vi "WriteCal.vi"(11 "Calibration table":T1={"version"=3, "table type"=25, "table size"=496, "full version"=67109889, "crc32"=2980334277, "baseline"=-55.153587, "model"=1, "fx left"=0.7094939, "fy left"=1.2617997, "px left"=0.49358395, "py left"=0.4803248, "py right"=0.4684578, "px right"=0.4979801, "fy right"=1.2668592, "fx right"=0.7124277, "k left"=[0.13808699, -0.41154006, 0.00043059044, 0.00047021545, 0.34858656], "k right"=[0.14090613, -0.42654052, -0.0003404384, 0.0005577445, 0.36482877], "RLeft"=[0.99998826, -0.004810224, 0.0006247892, 0.0048055355, 0.9999618, 0.0073000034, -0.00065988, -0.007296915, 0.9999732], "Rright"=[0.9999898, 0.00018351649, -0.0045086313, -0.00021641784, 0.99997336, -0.0072980113, 0.004507172, 0.007298913, 0.9999632], "uint8 reserved1"=[0, 0, 0, 0, 0, 0, 0, 0, 0, 0, 0, 0, 0, 0, 0, 0, 0, 0, 0, 0, 0, 0, 0, 0, 0, 0, 0, 0, 0, 0, 0, 0, 0, 0, 0, 0, 0, 0, 0, 0, 0, 0, 0, 0, 0, 0, 0, 0, 0, 0, 0, 0, 0, 0, 0, 0, 0, 0, 0, 0, 0, 0, 0, 0, 0, 0, 0, 0, 0, 0, 0, 0, 0, 0, 0, 0, 0, 0, 0, 0, 0, 0, 0, 0, 0, 0, 0, 0], "uint8 reserved2"=[0, 0, 0, 0, 0, 0, 0, 0, 0, 0, 0, 0, 0, 0, 0, 0, 0, 0, 0, 0, 0, 0, 0, 0, 0, 0, 0, 0, 0, 0, 0, 0, 0, 0, 0, 0, 0, 0, 0, 0, 0, 0, 0, 0, 0, 0, 0, 0, 0, 0, 0, 0, 0, 0, 0, 0, 0, 0, 0, 0, 0, 0, 0, 0], "1920x1080"=[1442.0812, 1442.0812, 949.4115, 513.11053], "1280x720"=[961.38745, 961.38745, 632.941, 342.07367], "640x480"=[640.925, 640.925, 315.29398, 228.04912], "848x480"=[640.925, 640.925, 419.29398, 228.04912], "640x360"=[480.69373, 480.69373, 316.4705, 171.03683], "424x240"=[320.4625, 320.4625, 209.64699, 114.02456], "320x240"=[320.4625, 320.4625, 157.64699, 114.02456], "480x270"=[360.5203, 360.5203, 237.35287, 128.27763], "1280x800"=[1068.2083, 1068.2083, 632.1567, 380.08188], "960x540"=[721.0406, 721.0406, 474.70575, 256.55527], "Reserved1"=[0.0, 0.0, 0.0, 0.0], "Reserved 2"=[0.0, 0.0, 0.0, 0.0]} {"crc32" format="%x"}) -> (2 "size":i32=512, 3 "Output array":u8[](array[numeric])=[197, 74, 164, 177, 240, 1, 0, 0, 1, 4, 0, 4, 197, 74, 164, 177, 100, 161, 53, 63, 167, 130, 161, 63, 9, 183, 252, 62, 34, 237, 245, 62, 173, 102, 13, 62, 97, 181, 210, 190, 223, 192, 225, 57, 64, 135, 246, 57, 240, 121, 178, 62, 169, 97, 54, 63, 113, 40, 162, 63, 63, 247, 254, 62, 179, 217, 239, 62, 178, 73, 16, 62, 133, 99, 218, 190, 222, 124, 178, 185, 154, 53, 18, 58, 214, 202, 186, 62, 59, 255, 127, 63, 21, 159, 157, 187, 229, 200, 35, 58, 193, 119, 157, 59, 127, 253, 127, 63, 222, 52, 239, 59, 204, 251, 44, 186, 246, 26, 239, 187, 62, 254, 127, 63, 85, 255, 127, 63, 85, 110, 64, 57, 36, 189, 147, 187, 57, 238, 98, 185, 65, 254, 127, 63, 40, 36, 239, 187, 230, 176, 147, 59, 184, 43, 239, 59, 151, 253, 127, 63, 70, 157, 92, 194, 1, 0, 0, 0, 0, 0, 0, 0, 0, 0, 0, 0, 0, 0, 0, 0, 0, 0, 0, 0, 0, 0, 0, 0, 0, 0, 0, 0, 0, 0, 0, 0, 0, 0, 0, 0, 0, 0, 0, 0, 0, 0, 0, 0, 0, 0, 0, 0, 0, 0, 0, 0, 0, 0, 0, 0, 0, 0, 0, 0, 0, 0, 0, 0, 0, 0, 0, 0, 0, 0, 0, 0, 0, 0, 0, 0, 0, 0, 0, 0, 0, 0, 0, 0, 0, 0, 0, 0, 0, 0, 0, 0, 153, 66, 180, 68, 153, 66, 180, 68, 86, 90, 109, 68, 19, 71, 0, 68, 204, 88, 112, 68, 204, 88, 112, 68, 57, 60, 30, 68, 110, 9, 171, 67, 51, 59, 32, 68, 51, 59, 32, 68, 161, 165, 157, 67, 147, 12, 100, 67, 51, 59, 32, 68, 51, 59, 32, 68, 161, 165, 209, 67, 147, 12, 100, 67, 204, 88, 240, 67, 204, 88, 240, 67, 57, 60, 158, 67, 110, 9, 43, 67, 51, 59, 160, 67, 51, 59, 160, 67, 161, 165, 81, 67, 147, 12, 228, 66, 51, 59, 160, 67, 51, 59, 160, 67, 161, 165, 29, 67, 147, 12, 228, 66, 153, 66, 180, 67, 153, 66, 180, 67, 86, 90, 109, 67, 19, 71, 0, 67, 170, 134, 133, 68, 170, 134, 133, 68, 7, 10, 30, 68, 123, 10, 190, 67, 153, 66, 52, 68, 153, 66, 52, 68, 86, 90, 237, 67, 19, 71, 128, 67, 0, 0, 0, 0, 0, 0, 0, 0, 0, 0, 0, 0, 0, 0, 0, 0, 0, 0, 0, 0, 0, 0, 0, 0, 0, 0, 0, 0, 0, 0, 0, 0, 0, 0, 0, 0, 0, 0, 0, 0, 0, 0, 0, 0, 0, 0, 0, 0, 0, 0, 0, 0, 0, 0, 0, 0, 0, 0, 0, 0, 0, 0, 0, 0, 0, 0, 0, 0, 0, 0, 0, 0, 0, 0, 0, 0, 0, 0, 0, 0, 0, 0, 0, 0, 0, 0, 0, 0, 0, 0, 0, 0, 0, 0, 0, 0] format="%x")   [LabVIEW 2017, in "libRealSense3.lvlib"]
uses:
  libRealSense3.lvlib
panel:
  out "input":u8[](array[numeric]) format="%x"
  out "Calibration table 2":T1={"version"=3, "table type"=25, "table size"=496, "full version"=67109889, "crc32"=2980334277, "baseline"=-55.153587, "model"=1, "fx left"=0.7094939, "fy left"=1.2617997, "px left"=0.49358395, "py left"=0.4803248, "py right"=0.4684578, "px right"=0.4979801, "fy right"=1.2668592, "fx right"=0.7124277, "k left"=[0.13808699, -0.41154006, 0.00043059044, 0.00047021545, 0.34858656], "k right"=[0.14090613, -0.42654052, -0.0003404384, 0.0005577445, 0.36482877], "RLeft"=[0.99998826, -0.004810224, 0.0006247892, 0.0048055355, 0.9999618, 0.0073000034, -0.00065988, -0.007296915, 0.9999732], "Rright"=[0.9999898, 0.00018351649, -0.0045086313, -0.00021641784, 0.99997336, -0.0072980113, 0.004507172, 0.007298913, 0.9999632], "uint8 reserved1"=[0, 0, 0, 0, 0, 0, 0, 0, 0, 0, 0, 0, 0, 0, 0, 0, 0, 0, 0, 0, 0, 0, 0, 0, 0, 0, 0, 0, 0, 0, 0, 0, 0, 0, 0, 0, 0, 0, 0, 0, 0, 0, 0, 0, 0, 0, 0, 0, 0, 0, 0, 0, 0, 0, 0, 0, 0, 0, 0, 0, 0, 0, 0, 0, 0, 0, 0, 0, 0, 0, 0, 0, 0, 0, 0, 0, 0, 0, 0, 0, 0, 0, 0, 0, 0, 0, 0, 0], "uint8 reserved2"=[0, 0, 0, 0, 0, 0, 0, 0, 0, 0, 0, 0, 0, 0, 0, 0, 0, 0, 0, 0, 0, 0, 0, 0, 0, 0, 0, 0, 0, 0, 0, 0, 0, 0, 0, 0, 0, 0, 0, 0, 0, 0, 0, 0, 0, 0, 0, 0, 0, 0, 0, 0, 0, 0, 0, 0, 0, 0, 0, 0, 0, 0, 0, 0], "1920x1080"=[1442.0812, 1442.0812, 949.4115, 513.11053], "1280x720"=[961.38745, 961.38745, 632.941, 342.07367], "640x480"=[640.925, 640.925, 315.29398, 228.04912], "848x480"=[640.925, 640.925, 419.29398, 228.04912], "640x360"=[480.69373, 480.69373, 316.4705, 171.03683], "424x240"=[320.4625, 320.4625, 209.64699, 114.02456], "320x240"=[320.4625, 320.4625, 157.64699, 114.02456], "480x270"=[360.5203, 360.5203, 237.35287, 128.27763], "1280x800"=[1068.2083, 1068.2083, 632.1567, 380.08188], "960x540"=[721.0406, 721.0406, 474.70575, 256.55527], "Reserved1"=[0.0, 0.0, 0.0, 0.0], "Reserved 2"=[0.0, 0.0, 0.0, 0.0]} {"crc32" format="%x"}
  out "New CRC output":u32=2980334277 format="%x"
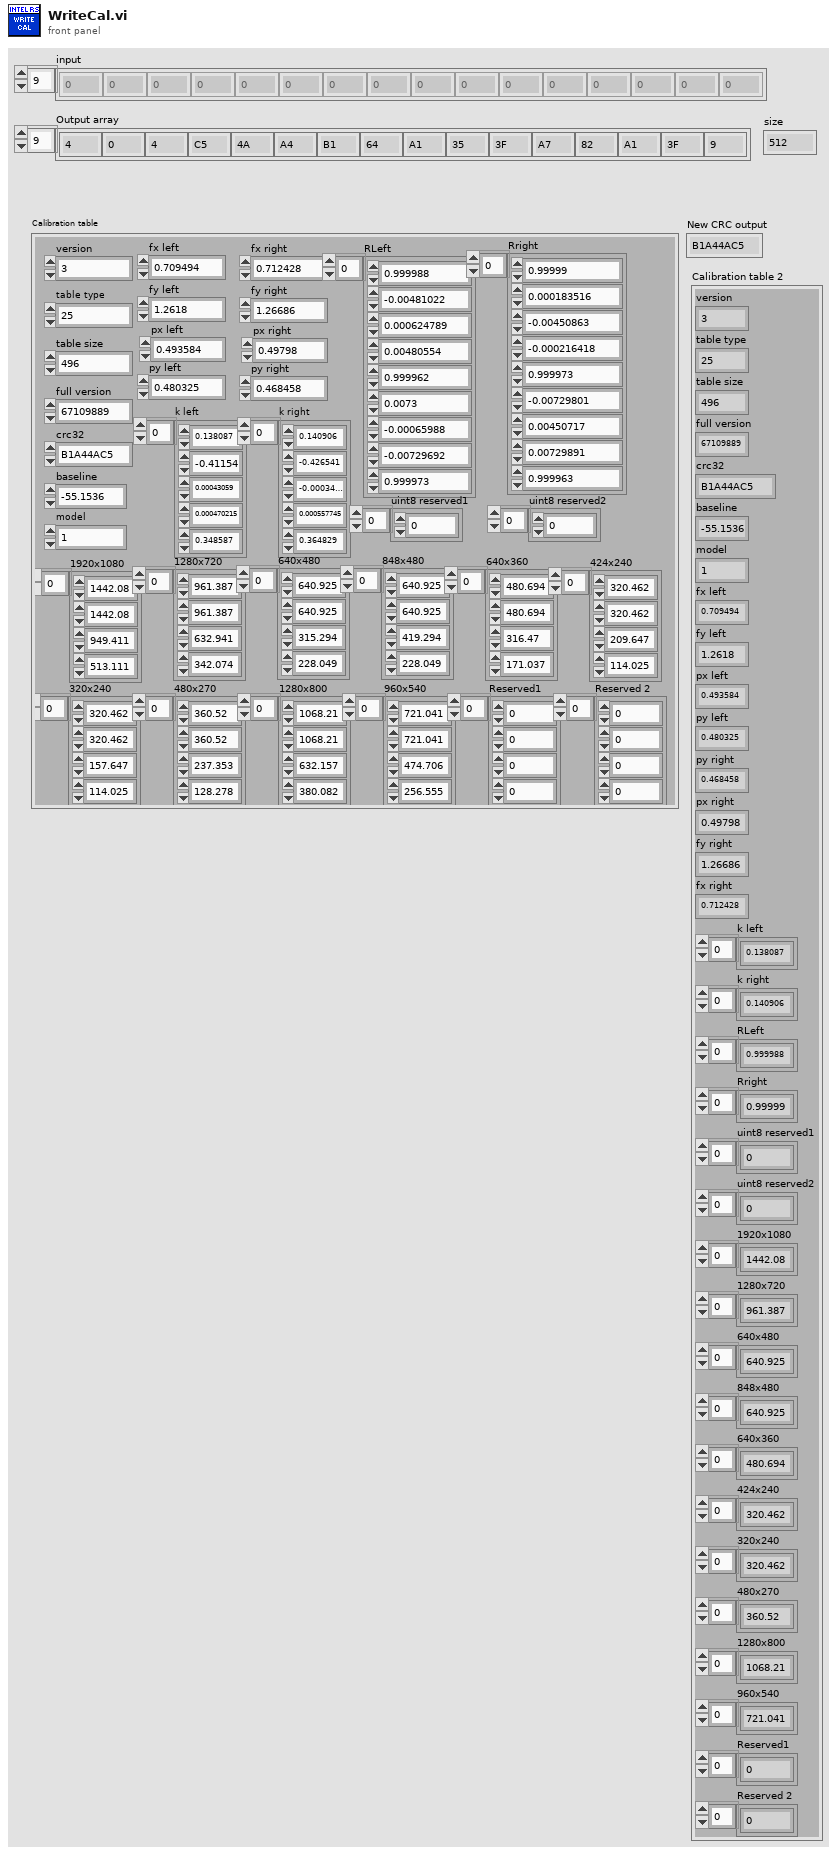
[diagram p1: front panel]
types:
  T1 = cluster{"version":u16, "table type":u16, "table size":u32, "full version":u32, "crc32":u32, "baseline":sgl, "model":u32, "fx left":sgl, "fy left":sgl, "px left":sgl, "py left":sgl, "py right":sgl, "px right":sgl, "fy right":sgl, "fx right":sgl, "k left":sgl[], "k right":sgl[], "RLeft":sgl[], "Rright":sgl[], "uint8 reserved1":u8[], "uint8 reserved2":u8[], "1920x1080":sgl[], "1280x720":sgl[], "640x480":sgl[], "848x480":sgl[], "640x360":sgl[], "424x240":sgl[], "320x240":sgl[], "480x270":sgl[], "1280x800":sgl[], "960x540":sgl[], "Reserved1":sgl[], "Reserved 2":sgl[]}
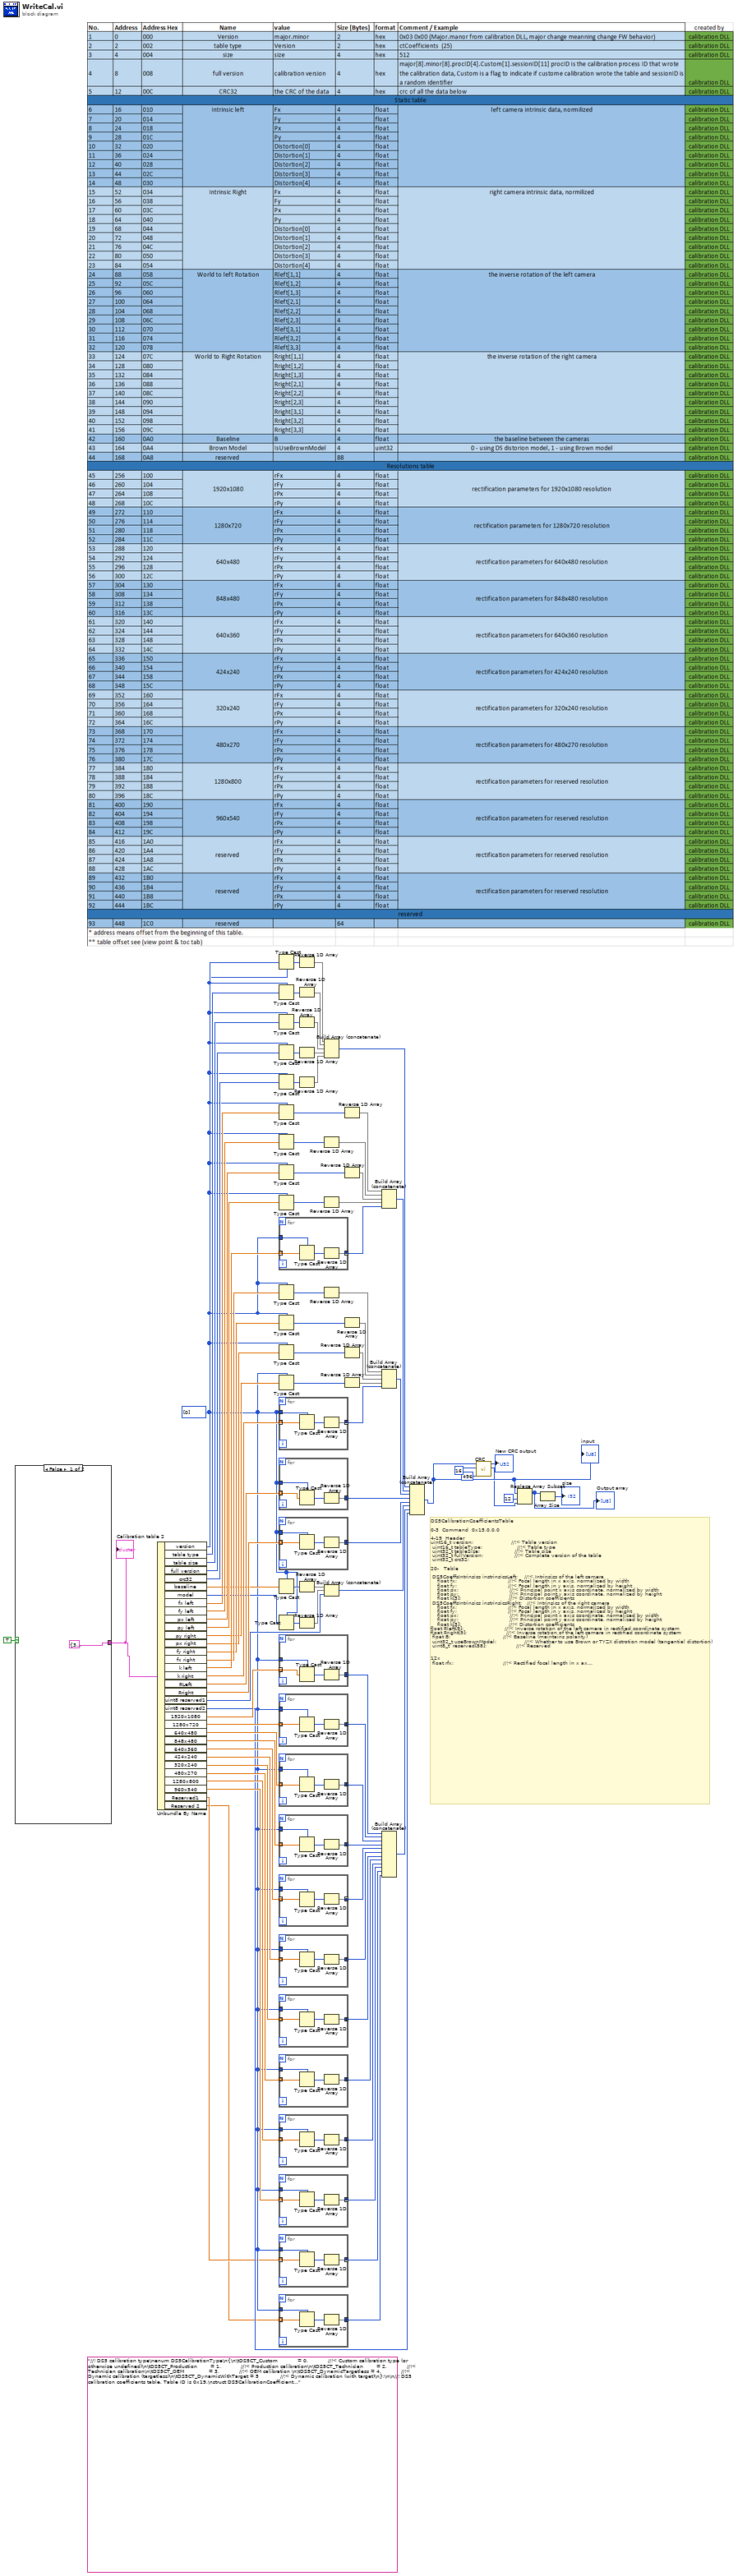
[diagram p0: block diagram]
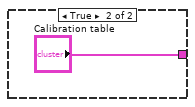
[diagram p2: hidden frame]
diagram:
  (unwired) "//! DS5 calibration type\nenum DS5CalibrationType\n{\n\tDS5CT_Custom            = 0,            //!< Custom calibration type (or otherwise undefined)\n\tDS5CT_Production        = 1,            //!< Production calibration\n\tDS5CT_Technician        = 2,            //!< Technician calibration\n\tDS5CT_OEM               = 3,            //!< OEM calibration \n\tDS5CT_DynamicTargetless = 4,            //!< Dynamic calibration (targetless)\n\tDS5CT_DynamicWithTarget = 5             //!< Dynamic calibration (with target)\n};\n\n//! DS5 calibration coefficients table. Table ID is 0x19.\nstruct DS5CalibrationCoefficientsTable\n{\n\tDS5CalibrationTableHeader header;       //!< Header\n\tDS5CalibrationCoefficients coeffs;      //!< Coefficients\n\tDS5CoeffsMode  modes[12];               //!< Rectified camera parameters. Each entry in the table corresponds to a resolution\n\tuint8_t  reserved2[64];                 //!< Reserved\n};\n\nstruct DS5CalibrationTableHeader\n{\n\tuint16_t version;                       //!< Table version\n\tuint16_t tableType;                     //!< Table type\n\tuint32_t tableSize;                     //!< Table size \n\tuint32_t fullVersion;                   //!< Complete version of the table\n\tuint32_t crc32;                         //!< CRC32 of the content\n};\n\nstruct DS5CalibrationCoefficients\n{\n\tDS5CoeffsIntrinsics instrinsicsLeft;    //!< Intrinsics of the left camera\n\tDS5CoeffsIntrinsics instrinsicsRight;   //!< Intrinsics of the right camera\n\tfloat Rleft[9];                         //!< Inverse rotation of the left camera in rectified coordinate system\n\tfloat Rright[9];                        //!< Inverse rotation of the left camera in rectified coordinate system\n\tfloat B;                                //!< Baseline (maintains polarity)\n\tuint32_t useBrownModel;                 //!< Whether to use Brown or TYZX distrotion model (tangential distortion)\n\tuint8_t  reserved[88];                  //!< Reserved\n};\n\nstruct DS5CoeffsMode\n{\n\tfloat rfx;                              //!< Rectified focal length in x axis\n\tfloat rfy;                              //!< Rectified focal length in y axis\n\tfloat rpx;                              //!< Rectified principal point x axis coordinate\n\tfloat rpy;                              //!< Rectified principal point y axis coordinate\n};\n\nstruct DS5CoeffsIntrinsics\n{\n\tfloat fx;                               //!< Focal length in x axis, normalized by width\n\tfloat fy;                               //!< Focal length in y axis, normalized by height\n\tfloat px;                               //!< Principal point x axis coordinate, normalized by width\n\tfloat py;                               //!< Principal point y axis coordinate, normalized by height\n\tfloat k[5];                             //!< Distortion coefficients\n};\n\n/** \\brief Distortion model: defines how pixel coordinates should be mapped to sensor coordinates. */\ntypedef enum rs2_distortion\n{\n    RS2_DISTORTION_NONE                  , /**< Rectilinear images. No distortion compensation required. */\n    RS2_DISTORTION_MODIFIED_BROWN_CONRADY, /**< Equivalent to Brown-Conrady distortion, except that tangential distortion is applied to radially distorted points */\n    RS2_DISTORTION_INVERSE_BROWN_CONRADY , /**< Equivalent to Brown-Conrady distortion, except undistorts image instead of distorting it */\n    RS2_DISTORTION_FTHETA                , /**< F-Theta fish-eye distortion model */\n    RS2_DISTORTION_BROWN_CONRADY         , /**< Unmodified Brown-Conrady distortion model */\n    RS2_DISTORTION_COUNT                 , /**< Number of enumeration values. Not a valid input: intended to be used in for-loops. */\n} rs2_distortion;\n\n//! DS5 recitifed resolution index\nenum DS5CoeffsModeIndex\n{\n\tDS5M_1920_1080 = 0,                     //!< 1920x1080 rectified resolution (R8L8 only)\n\tDS5M_1280_720  = 1,                     //!< 1280x720 rectified resolution\n\tDS5M_640_480   = 2,                     //!< 640x480 rectified resolution\n\tDS5M_848_480   = 3,                     //!< 848x480 rectified resolution\n\tDS5M_640_360   = 4,                     //!< 640x360 rectified resolution\n\tDS5M_424_240   = 5,                     //!< 424x240 rectified resolution\n\tDS5M_320_240   = 6,                     //!< 320x240 rectified resolution\n\tDS5M_480_270   = 7,                     //!< 480x270 rectified resolution\n\tDS5M_1280_800  = 8,                     //!< 1280x800 rectified resolution (R8L8 only)\n\tDS5M_960_540   = 9                      //!< 960x540 rectified resolution\n};"
  w14 = u8[] [0]
  # "DS5CalibrationCoefficientsTable\n\n0-3  Command  0x15,0,0,0\n\n4-19\t Header\nuint16_t version;                       //!< Table version\n\tuint16_t tableType;                     //!< Table type\n\tuint32_t tableSize;                     //!< Table size \n\tuint32_t fullVersion;                   //!< Complete version of the table\n\tuint32_t crc32; \n\n20-   Table\n\n\tDS5CoeffsIntrinsics instrinsicsLeft;    //!< Intrinsics of the left camera\n   \tfloat fx;                               //!< Focal length in x axis, normalized by width\n   \tfloat fy;                               //!< Focal length in y axis, normalized by height\n\t   float px;                               //!< Principal point x axis coordinate, normalized by width\n\t   float py;                               //!< Principal point y axis coordinate, normalized by height\n\t   float k[5];                             //!< Distortion coefficients\n\tDS5CoeffsIntrinsics instrinsicsRight;   //!< Intrinsics of the right camera\n   \tfloat fx;                               //!< Focal length in x axis, normalized by width\n   \tfloat fy;                               //!< Focal length in y axis, normalized by height\n\t   float px;                               //!< Principal point x axis coordinate, normalized by width\n\t   float py;                               //!< Principal point y axis coordinate, normalized by height\n\t   float k[5];                             //!< Distortion coefficients\t\nfloat Rleft[9];                         //!< Inverse rotation of the left camera in rectified coordinate system\nfloat Rright[9];                        //!< Inverse rotation of the left camera in rectified coordinate system\n\tfloat B;                                //!< Baseline (maintains polarity)\n\tuint32_t useBrownModel;                 //!< Whether to use Brown or TYZX distrotion model (tangential distortion)\n\tuint8_t  reserved[88];                  //!< Reserved\n\n\n12x \n\tfloat rfx;                              //!< Rectified focal length in x axis\n\tfloat rfy;                              //!< Rectified focal length in y axis\n\tfloat rpx;                              //!< Rectified principal point x axis coordinate\n\tfloat rpy;                              //!< Rectified principal point y axis coordinate\n\n64x reserved"
  n1 = case shown="False" TRUE {
    tunnel: [T1 {"version"=3, "table type"=60479, "table size"=496, "full version"=67109888, "crc32"=3963612841, "baseline"=-54.831806, "model"=1, "fx left"=917.7658, "fy left"=915.4345, "px left"=631.39185, "py left"=376.6227, "py right"=364.3492, "px right"=651.2822, "fy right"=921.49005, "fx right"=923.5849, "k left"=[0.13533829, -0.40519878, 0.0008784002, -0.0011180333, 0.3588802], "k right"=[0.12740475, -0.39763576, 0.00037952562, -0.0022863527, 0.35284942], "RLeft"=[0.9999986, 0.0009555143, -0.001359244, -0.0009574645, 0.9999985, -0.001434832, 0.001357871, 0.0014361315, 0.99999803], "Rright"=[0.99998456, -0.0019937593, -0.0051888847, 0.002001206, 0.99999696, 0.0014302958, 0.0051860176, -0.0014406577, 0.9999855], "uint8 reserved1"=[0, 0, 0, 0, 0, 0, 0, 0, 0, 0, 0, 0, 0, 0, 0, 0, 0, 0, 0, 0, 0, 0, 0, 0, 0, 0, 0, 0, 0, 0, 0, 0, 0, 0, 0, 0, 0, 0, 0, 0, 0, 0, 0, 0, 0, 0, 0, 0, 0, 0, 0, 0, 0, 0, 0, 0, 0, 0, 0, 0, 0, 0, 0, 0, 0, 0, 0, 0, 0, 0, 0, 0, 0, 0, 0, 0, 0, 0, 0, 0, 0, 0, 0, 0, 0, 0, 0, 0], "uint8 reserved2"=[0, 0, 0, 0, 0, 0, 0, 0, 0, 0, 0, 0, 0, 0, 0, 0, 0, 0, 0, 0, 0, 0, 0, 0, 0, 0, 0, 0, 0, 0, 0, 0, 0, 0, 0, 0, 0, 0, 0, 0, 0, 0, 0, 0, 0, 0, 0, 0, 0, 0, 0, 0, 0, 0, 0, 0, 0, 0, 0, 0, 0, 0, 0, 0], "1920x1080"=[1428.9095, 1428.9095, 951.85925, 556.0496], "1280x720"=[952.6064, 952.6064, 634.5728, 370.69974], "640x480"=[635.0709, 635.0709, 316.38187, 247.13316], "848x480"=[635.0709, 635.0709, 420.38187, 247.13316], "640x360"=[476.3032, 476.3032, 317.2864, 185.34987], "424x240"=[317.53546, 317.53546, 210.19093, 123.56658], "320x240"=[317.53546, 317.53546, 158.19093, 123.56658], "480x270"=[357.2274, 357.2274, 237.96481, 139.0124], "1280x800"=[1058.4515, 1058.4515, 633.9698, 411.8886], "960x540"=[714.4548, 714.4548, 475.92963, 278.0248], "Reserved1"=[714.4548, 714.4548, 475.92963, 278.0248], "Reserved 2"=[714.4548, 714.4548, 475.92963, 278.0248]} ("Calibration table 2") "Calibration table"] -> w3
    frame False {
    }
    frame True {
    }
  }
  "Calibration table 2" <- w3
  n2 = Unbundle By Name(w3) -> ("version"=w94:u16, "table type"=w92:u16, "table size"=w90:u32, "full version"=w85:u32, "crc32"=w83:u32, "baseline"=w44:sgl, "model"=w42:u32, "fx left"=w79:sgl, "fy left"=w77:sgl, "px left"=w76:sgl, "py left"=w75:sgl, "py right"=w52:sgl, "px right"=w53:sgl, "fy right"=w54:sgl, "fx right"=w55:sgl, "k left"=w65:sgl[], "k right"=w51:sgl[], "RLeft"=w49:sgl[], "Rright"=w48:sgl[], "uint8 reserved1"=w37:u8[], "uint8 reserved2"=w15:u8[], "1920x1080"=w38:sgl[], "1280x720"=w36:sgl[], "640x480"=w35:sgl[], "848x480"=w34:sgl[], "640x360"=w33:sgl[], "424x240"=w32:sgl[], "320x240"=w31:sgl[], "480x270"=w30:sgl[], "1280x800"=w29:sgl[], "960x540"=w28:sgl[], "Reserved1"=w5:sgl[], "Reserved 2"=w4:sgl[])
  n3 = Type Cast(type=w14, x=w94) -> (*(type *) &x=w95:u8[])
  n4 = Type Cast(type=w14, x=w92) -> (*(type *) &x=w93:u8[])
  n5 = Type Cast(type=w14, x=w90) -> (*(type *) &x=w91:u8[])
  n6 = Type Cast(type=w14, x=w85) -> (*(type *) &x=w86:u8[])
  n7 = Type Cast(type=w14, x=w83) -> (*(type *) &x=w82:u8[])
  n8 = Type Cast(type=w14, x=w79) -> (*(type *) &x=w80:u8[])
  n9 = Type Cast(type=w14, x=w77) -> (*(type *) &x=w74:u8[])
  n10 = Type Cast(type=w14, x=w76) -> (*(type *) &x=w73:u8[])
  n11 = Type Cast(type=w14, x=w75) -> (*(type *) &x=w72:u8[])
  n12 = for {
    tunnel: [w100] -> w66 mode=concatenating
    tunnel: w65 -> [w99] mode=indexing
    tunnel: w14 -> [w98]
    n13 = Type Cast(type=w98, x=w99) -> (*(type *) &x=w101:u8[])
    n14 = Reverse 1D Array(array=w101) -> (reversed array=w100:u8[])
  }
  n15 = Type Cast(type=w14, x=w55) -> (*(type *) &x=w56:u8[])
  n16 = Type Cast(type=w14, x=w54) -> (*(type *) &x=w58:u8[])
  n17 = Type Cast(type=w14, x=w53) -> (*(type *) &x=w59:u8[])
  n18 = Type Cast(type=w14, x=w52) -> (*(type *) &x=w60:u8[])
  n19 = for {
    tunnel: [w104] -> w64 mode=concatenating
    tunnel: w14 -> [w103]
    tunnel: w51 -> [w102] mode=indexing
    n20 = Type Cast(type=w103, x=w102) -> (*(type *) &x=w105:u8[])
    n21 = Reverse 1D Array(array=w105) -> (reversed array=w104:u8[])
  }
  n22 = for {
    tunnel: [w108] -> w47 mode=concatenating
    tunnel: w14 -> [w107]
    tunnel: w49 -> [w106] mode=indexing
    n23 = Type Cast(type=w107, x=w106) -> (*(type *) &x=w109:u8[])
    n24 = Reverse 1D Array(array=w109) -> (reversed array=w108:u8[])
  }
  n25 = for {
    tunnel: [w112] -> w46 mode=concatenating
    tunnel: w14 -> [w111]
    tunnel: w48 -> [w110] mode=indexing
    n26 = Type Cast(type=w111, x=w110) -> (*(type *) &x=w113:u8[])
    n27 = Reverse 1D Array(array=w113) -> (reversed array=w112:u8[])
  }
  n28 = Type Cast(type=w14, x=w44) -> (*(type *) &x=w45:u8[])
  n29 = Type Cast(type=w14, x=w42) -> (*(type *) &x=w43:u8[])
  n30 = for {
    tunnel: [w116] -> w27 mode=concatenating
    tunnel: w14 -> [w115]
    tunnel: w38 -> [w114] mode=indexing
    n31 = Type Cast(type=w115, x=w114) -> (*(type *) &x=w117:u8[])
    n32 = Reverse 1D Array(array=w117) -> (reversed array=w116:u8[])
  }
  n33 = for {
    tunnel: [w120] -> w26 mode=concatenating
    tunnel: w14 -> [w119]
    tunnel: w36 -> [w118] mode=indexing
    n34 = Type Cast(type=w119, x=w118) -> (*(type *) &x=w121:u8[])
    n35 = Reverse 1D Array(array=w121) -> (reversed array=w120:u8[])
  }
  n36 = for {
    tunnel: [w124] -> w25 mode=concatenating
    tunnel: w14 -> [w123]
    tunnel: w35 -> [w122] mode=indexing
    n37 = Type Cast(type=w123, x=w122) -> (*(type *) &x=w125:u8[])
    n38 = Reverse 1D Array(array=w125) -> (reversed array=w124:u8[])
  }
  n39 = for {
    tunnel: [w128] -> w24 mode=concatenating
    tunnel: w14 -> [w127]
    tunnel: w34 -> [w126] mode=indexing
    n40 = Type Cast(type=w127, x=w126) -> (*(type *) &x=w129:u8[])
    n41 = Reverse 1D Array(array=w129) -> (reversed array=w128:u8[])
  }
  n42 = for {
    tunnel: [w132] -> w23 mode=concatenating
    tunnel: w14 -> [w131]
    tunnel: w33 -> [w130] mode=indexing
    n43 = Type Cast(type=w131, x=w130) -> (*(type *) &x=w133:u8[])
    n44 = Reverse 1D Array(array=w133) -> (reversed array=w132:u8[])
  }
  n45 = for {
    tunnel: [w136] -> w22 mode=concatenating
    tunnel: w14 -> [w135]
    tunnel: w32 -> [w134] mode=indexing
    n46 = Type Cast(type=w135, x=w134) -> (*(type *) &x=w137:u8[])
    n47 = Reverse 1D Array(array=w137) -> (reversed array=w136:u8[])
  }
  n48 = for {
    tunnel: [w140] -> w21 mode=concatenating
    tunnel: w14 -> [w139]
    tunnel: w31 -> [w138] mode=indexing
    n49 = Type Cast(type=w139, x=w138) -> (*(type *) &x=w141:u8[])
    n50 = Reverse 1D Array(array=w141) -> (reversed array=w140:u8[])
  }
  n51 = for {
    tunnel: [w144] -> w20 mode=concatenating
    tunnel: w14 -> [w143]
    tunnel: w30 -> [w142] mode=indexing
    n52 = Type Cast(type=w143, x=w142) -> (*(type *) &x=w145:u8[])
    n53 = Reverse 1D Array(array=w145) -> (reversed array=w144:u8[])
  }
  n54 = for {
    tunnel: [w148] -> w19 mode=concatenating
    tunnel: w14 -> [w147]
    tunnel: w29 -> [w146] mode=indexing
    n55 = Type Cast(type=w147, x=w146) -> (*(type *) &x=w149:u8[])
    n56 = Reverse 1D Array(array=w149) -> (reversed array=w148:u8[])
  }
  n57 = for {
    tunnel: [w152] -> w18 mode=concatenating
    tunnel: w14 -> [w151]
    tunnel: w28 -> [w150] mode=indexing
    n58 = Type Cast(type=w151, x=w150) -> (*(type *) &x=w153:u8[])
    n59 = Reverse 1D Array(array=w153) -> (reversed array=w152:u8[])
  }
  n60 = for {
    tunnel: [w156] -> w13 mode=concatenating
    tunnel: w14 -> [w155]
    tunnel: w5 -> [w154] mode=indexing
    n61 = Type Cast(type=w155, x=w154) -> (*(type *) &x=w157:u8[])
    n62 = Reverse 1D Array(array=w157) -> (reversed array=w156:u8[])
  }
  n63 = for {
    tunnel: [w160] -> w12 mode=concatenating
    tunnel: w14 -> [w159]
    tunnel: w4 -> [w158] mode=indexing
    n64 = Type Cast(type=w159, x=w158) -> (*(type *) &x=w161:u8[])
    n65 = Reverse 1D Array(array=w161) -> (reversed array=w160:u8[])
  }
  n66 = Reverse 1D Array(array=w95) -> (reversed array=w89:u8[])
  n67 = Reverse 1D Array(array=w93) -> (reversed array=w88:u8[])
  n68 = Reverse 1D Array(array=w91) -> (reversed array=w87:u8[])
  n69 = Reverse 1D Array(array=w86) -> (reversed array=w84:u8[])
  n70 = Reverse 1D Array(array=w82) -> (reversed array=w81:u8[])
  n71 = Reverse 1D Array(array=w45) -> (reversed array=w41:u8[])
  n72 = Reverse 1D Array(array=w43) -> (reversed array=w40:u8[])
  n73 = Build Array (concatenate)(w89, w88, w87, w84, w81) -> (w68:u8[])
  n74 = Reverse 1D Array(array=w74) -> (reversed array=w71:u8[])
  n75 = Reverse 1D Array(array=w72) -> (reversed array=w69:u8[])
  n76 = Reverse 1D Array(array=w56) -> (reversed array=w57:u8[])
  n77 = Build Array (concatenate)(w41, w40, w37) -> (w39:u8[])
  n78 = Reverse 1D Array(array=w80) -> (reversed array=w78:u8[])
  n79 = Reverse 1D Array(array=w73) -> (reversed array=w70:u8[])
  n80 = Reverse 1D Array(array=w58) -> (reversed array=w61:u8[])
  n81 = Reverse 1D Array(array=w59) -> (reversed array=w62:u8[])
  n82 = Reverse 1D Array(array=w60) -> (reversed array=w63:u8[])
  n83 = Build Array (concatenate)(w78, w71, w70, w69, w66) -> (w67:u8[])
  n84 = Build Array (concatenate)(w57, w61, w62, w63, w64) -> (w50:u8[])
  n85 = Build Array (concatenate)(w27, w26, w25, w24, w23, w22, w21, w20, w19, w18, w13, w12) -> (w17:u8[])
  n86 = Build Array (concatenate)(w68, w67, w50, w47, w46, w39, w17, w15) -> (w9:u8[])
  "input" <- w9
  n87 = call "CRC.vi"("length"=496, "index"=16, "DS5CalibrationCoefficientsTable"=w9) -> ("CRC array"=w7:u8[], "CRC output"=→"New CRC output":u32)  [unwired: 7 in]
  n88 = Replace Array Subset(array=w9, new element=w7, index=12) -> (w6:u8[])
  "Output array" <- w6
  n89 = Array Size(array=w6) -> (size(s)=→"size":i32)
